vi "2D STR Array_Sort and Delete Repeating Sells.vi"(2 "2D STRL Array.In":string[][](array[string]), 4 "index":i32) -> (6 "2D STR Array.Out":string[][](array[string]))   [LabVIEW 2020]
uses:
  71fc4bf8-ae4c-47e9-baa3-e4ad21f60e08.vi
  <vilib>/Array/Sort 2D Array - Pop Stack.vi
  <vilib>/Array/Sort 2D Array - Push Stack.vi
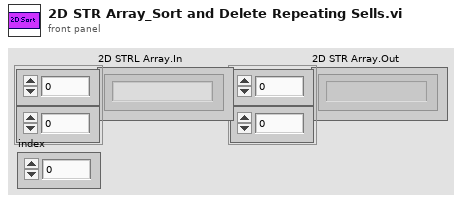
[diagram p1: front panel]
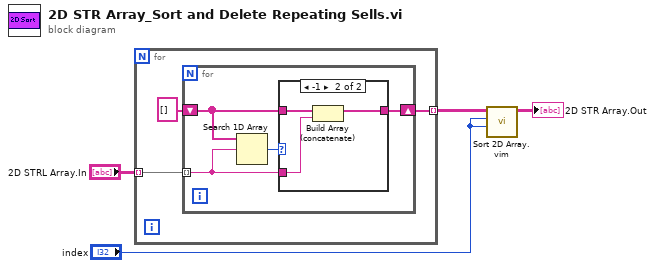
[diagram p0: block diagram]
diagram:
  n1 = for {
    tunnel: [w7] -> w3 mode=indexing
    tunnel: "2D STRL Array.In" -> [w5] mode=indexing
    n2 = for {
      tunnel: w5 -> [w9] mode=indexing
      shift-right: [w8] -> w7
      shift-left: string[] [] ("sorted array") -> [w10]
      n3 = Search 1D Array(1D array=w10, element=w9) -> (index of element=w11:i32)  [unwired: 1 in]
      n4 = case shown="-1" w11 {
        tunnel: w10 -> [w12 w15]
        tunnel: w9 -> [_ w14]
        tunnel: [w12 w13] -> w8
        frame 0, Default {
        }
        frame -1 {
          n5 = Build Array (concatenate)(w15, w14) -> (w13:string[])
        }
      }
    }
  }
  n6 = call "Sort 2D Array.vim"("index"="index", "dimension to index (column)"="index", "2D array"=w3) -> ("sorted 2D array"=→"2D STR Array.Out":string[][])  [unwired: 7 in, 1 out]
